vi "Fit_Poly2Disc_fcn.vi"(3 "output control":T1, 4 "data":T2, 5 "X":dbl[](array[numeric])) -> (0 "error out":errorcluster, 1 "gradient":dbl[](array[numeric]), 2 "f(X)":dbl)   [LabVIEW 2022 SP3]
doc: "This template is the starting point for creating an objectivel function to be passed to the Unconstrained Optimization.vi."
uses:
  <vilib>/gmath/NumericalOptimization/objective function data.ctl
  Displacement Data.ctl
  <vilib>/Analysis/baseanly.llb/Quick Scale 1D.vi
  <vilib>/Analysis/baseanly.llb/Scale 1D.vi
  <vilib>/Analysis/baseanly.llb/Mean (DBL).vi
  <vilib>/Analysis/NI_AALBase.lvlib
  <vilib>/Analysis/NI_AALPro.lvlib
  <vilib>/gmath/NI_Gmath.lvlib
panel:
  in  "Graph?":bool
  out "Displacement Graph":cluster{"Rc":dbl[], "Xd(t,r)":dbl[]}[](graph)
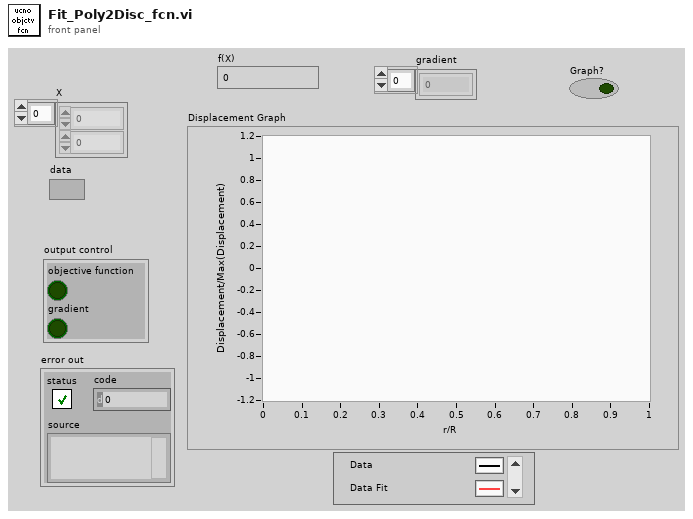
[diagram p1: front panel]
types:
  T1 = cluster{"objective function":bool, "gradient":bool}
  T2 = typedef "NI_Gmath.lvlib/objective function data.ctl" = variant
  T3 = typedef "Displacement Data.ctl" = cluster{"Xd(t,r)":dbl[][], "Rc":dbl[]}
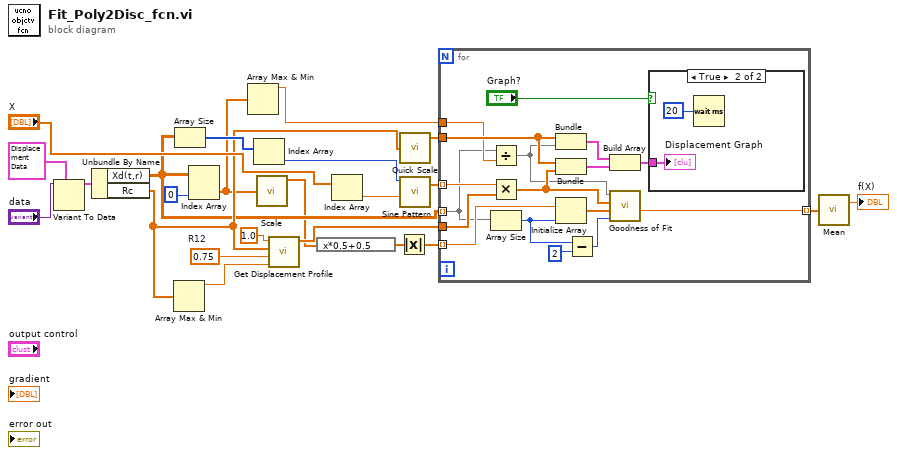
[diagram p0: block diagram]
diagram:
  w14 = 0.75  # R12
  n1 = Variant To Data(type=T3 {"Xd(t,r)"=array25x40[1000 elements], "Rc"=[-10.5, -9.5, -8.5, -7.5, -6.5, -5.5, -4.5, -3.5, -2.5, -1.5, -19.5, -0.5, 0.5, 1.5, 2.5, 3.5, 4.5, 5.5, 6.5, 7.5, 8.5, -18.5, 9.5, 10.5, 11.5, 12.5, 13.5, 14.5, 15.5, 16.5, 17.5, 18.5, -17.5, 19.5, -16.5, -15.5, -14.5, -13.5, -12.5, -11.5]} ("Displacement Data"), Variant="data") -> (data=w19:T3)  [unwired: 1 in, 1 out]
  n2 = Unbundle By Name(w19) -> ("Xd(t,r)"=w10:dbl[][], "Rc"=w11:dbl[])
  n3 = Array Max & Min(array=w11) -> (max value=w15:dbl)  [unwired: 3 out]
  n4 = Array Size(array=w10) -> (size(s)=w18:i32[])
  n5 = Index Array(array=w10, index (col)=0 ("disabled index (col)")) -> (element=w2:dbl[])  [unwired: 1 in]
  n6 = Array Max & Min(array=w2) -> (max value=w1:dbl)  [unwired: 3 out]
  n7 = Index Array(array=w18) -> (element=w17:i32)  [unwired: 1 in]
  n8 = call-poly <vilib>:"Scale.vi"("X"=w2) -> ("Y=(X-offset)/scale"=w9:dbl[])  [unwired: 3 out]
  n9 = call "Get Displacement Profile.vi"("R2"=w15, "R12"=w14, "r"=w11, "xd'"=1.0) -> ("xd (r)"=w12:dbl[])  [unwired: 7 in]
  n10 = expression code="x*0.5+0.5"(w9) -> (w8:dbl[])
  n11 = Index Array(array="X") -> (element=w22:dbl)  [unwired: 1 in]
  n12 = Absolute Value(x=w8) -> (abs(x)=w7:dbl[])
  n13 = call-poly <vilib>:"Quick Scale.vi"("X"=w11) -> ("Y[i]=X[i]/Max|X|"=w4:dbl[])  [unwired: 2 out]
  n14 = call <vilib>:"Sine Pattern.vi"("phase(degrees)"=w22, "samples"=w17) -> ("Sinusoidal Pattern"=w13:dbl[])  [unwired: 2 in, 1 out]
  n15 = for {
    tunnel: w13 -> [w40] mode=indexing
    tunnel: w12 -> [w39]
    tunnel: w4 -> [w27]
    tunnel: w10 -> [w25] mode=indexing
    tunnel: [w31] -> w6 mode=indexing
    tunnel: w7 -> [w30] mode=indexing
    tunnel: w1 -> [w26]
    n16 = Divide(x=w25, y=w26) -> (x/y=w24:dbl[])
    n17 = Multiply(x=w40, y=w39) -> (x*y=w28:dbl[])
    n18 = Array Size(array=w25) -> (size(s)=w33:i32)
    n19 = Bundle("Y[i]=X[i]/Max|X|"=w27, w24) -> (w38:cluster{"Y[i]=X[i]/Max|X|":dbl[], dbl[]})  [unwired: 1 in]
    n20 = Bundle("Y[i]=X[i]/Max|X|"=w27, w28) -> (w37:cluster{"Y[i]=X[i]/Max|X|":dbl[], dbl[]})  [unwired: 1 in]
    n21 = Initialize Array(w30, w33) -> (w34:dbl[])
    n22 = Subtract(x=w33, y=2) -> (x-y=w29:i32)
    n23 = Build Array(w38, w37) -> (w36:cluster{"Y[i]=X[i]/Max|X|":dbl[], dbl[]}[])
    n24 = call <vilib>:"Goodness of Fit.vi"("degree of freedom"=w29, "Weight"=w34, "Best Fit"=w28, "Y"=w24) -> ("RMSE"=w31:dbl)  [unwired: 4 in, 3 out]
    n25 = case shown="True" "Graph?" {
      tunnel: w36 -> [_ w42]
      frame False {
      }
      frame True {
        n26 = Wait (ms)(milliseconds to wait=u32 20) -> ()  [unwired: 1 out]
        "Displacement Graph" <- w42
      }
    }
  }
  n27 = call-poly <vilib>:"Mean.vi"("X"=w6) -> ("mean"=→"f(X)":dbl)  [unwired: 1 out]
